vi "SetServiceRequestEnableRegister.vi"(8 "Error In":errorcluster, 10 "Service Request Enable Register":bool[](array[boolean])=[FALSE, FALSE, FALSE, FALSE, FALSE, FALSE, FALSE, FALSE], 11 "Keithley 2602 In":refnum<visa-resource-name>) -> (0 "Error Out":errorcluster, 3 "Keithley 2602 Out":refnum<visa-resource-name>)   [LabVIEW 2012, in "Keithley-2602.lvlib"]
uses:
  Keithley-2602.lvlib
panel:
  # "MSB"
  # "EAV"
  # "MAV"
  # "RQS"
  # "SSB"
  # "QSB"
  # "ESB"
  # "OSB"
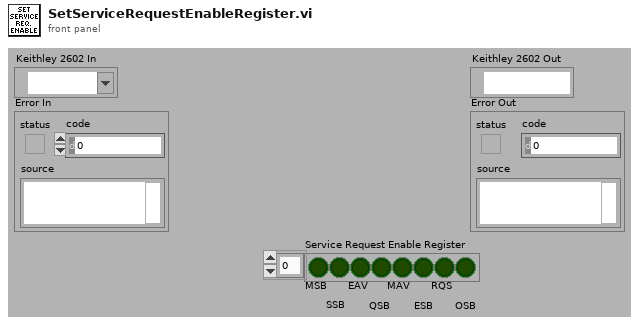
[diagram p1: front panel]
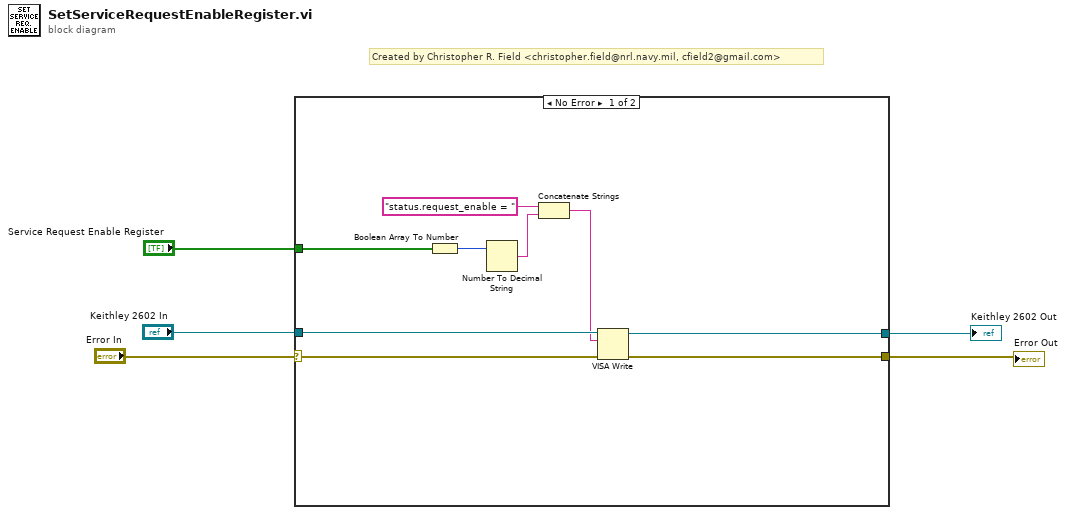
[diagram p0: block diagram]
diagram:
  # "Created by Christopher R. Field <christopher.field@nrl.navy.mil, cfield2@gmail.com>"
  n1 = case shown="No Error" "Error In" {
    selector: "Error In" -> [w6 w15]
    tunnel: "Keithley 2602 In" -> [w14 w16]
    tunnel: "Service Request Enable Register" -> [w13 _]
    tunnel: [w8 w16] -> w3
    tunnel: [w7 w15] -> w2
    frame No Error {
      n2 = Boolean Array To Number(Boolean array=w13) -> (number=w12:u32)
      n3 = Number To Decimal String(number=w12) -> (decimal integer string=w10:string)  [unwired: 1 in]
      n4 = Concatenate Strings("status.request_enable = ", w10) -> (w9:string)
      n5 = VISA Write(VISA resource name=w14, write buffer=w9, error in (no error)=w6) -> (VISA resource name out=w8:refnum<visa-resource-name>, error out=w7:errorcluster)  [unwired: 1 out]
    }
    frame Error {
    }
  }
  "Keithley 2602 Out" <- w3
  "Error Out" <- w2
